vi "CAN_ParamShow.vi"(10 "DevType":u16, 11 "param":T2[](array[typedef]) {"ACR0" format="%x"}) -> ()   [LabVIEW 2011]
uses:
  VIs/Param.ctl
  VIs/Baud rate Self Define.ctl
panel:
  out "br_selfdef":T1={"BAUD"=0, "SJW"=1, "BRP"=1, "SAM"=0, "PHS2_SEL"=0, "SYN(nouse)"=1, "PRSEG"=1, "PHSEG1"=1, "PHSEG2"=1} {"PHSEG2" items=["CAN_BIT_1TQ"=1, "CAN_BIT_2TQ"=2, "CAN_BIT_3TQ"=3, "CAN_BIT_4TQ"=4, "CAN_BIT_5TQ"=5, "CAN_BIT_6TQ"=6, "CAN_BIT_7TQ"=7, "CAN_BIT_8TQ"=8]; "PHSEG1" items=["CAN_BIT_1TQ"=1, "CAN_BIT_2TQ"=2, "CAN_BIT_3TQ"=3, "CAN_BIT_4TQ"=4, "CAN_BIT_5TQ"=5, "CAN_BIT_6TQ"=6, "CAN_BIT_7TQ"=7, "CAN_BIT_8TQ"=8]; "PRSEG" items=["CAN_BIT_1TQ"=1, "CAN_BIT_2TQ"=2, "CAN_BIT_3TQ"=3, "CAN_BIT_4TQ"=4, "CAN_BIT_5TQ"=5, "CAN_BIT_6TQ"=6, "CAN_BIT_7TQ"=7, "CAN_BIT_8TQ"=8]; "PHS2_SEL" items=["由相位缓冲段1时间指定", "可编程"]; "SAM" items=["采样一次", "采样三次"]; "BRP" items=["1"=1, "2"=2, "3"=3, "4"=4, "5"=5, "6"=6, "7"=7, "8"=8, "9"=9, "10"=10, "11"=11, "12"=12, "13"=13, "14"=14, "15"=15, "16"=16, "17"=17, "18"=18, "19"=19, "20"=20, "21"=21, "22"=22, "23"=23, "24"=24, "25"=25, "26"=26, "27"=27, "28"=28, "29"=29, "30"=30, "31"=31, "32"=32, "33"=33, "34"=34, "35"=35, "36"=36, "37"=37, "38"=38, "39"=39, "40"=40, "41"=41, "42"=42, "43"=43, "44"=44, "45"=45, "46"=46, "47"=47, "48"=48, "49"=49, "50"=50, "51"=51, "52"=52, "53"=53, "54"=54, "55"=55, "56"=56, "57"=57, "58"=58, "59"=59, "60"=60, "61"=61, "62"=62, "63"=63, "64"=64]; "SJW" items=["1TQ"=1, "2TQ"=2, "3TQ"=3, "4TQ"=4]; "SYN(nouse)" items=["CAN_BIT_1TQ"=1]}
  out "Filter":u8(ring)=3 caption="滤波方式：" items=["接收所有类型"=1, "只收标准帧"=2, "只收扩展帧"=3]
  out "屏蔽码":u32=4294967295 caption="过滤屏蔽码:" format="%08x"
  out "验收码":u32=2147483648 caption="过滤验收码:" format="%08x"
  out "工作模式":u16(ring)=1 items=["正常工作", "仅监帧听模式", "自测模试（环回模式）"]
  out "br":u32(ring)=8 caption="波特率:" items=["Self Define", "5k bps", "10k bps", "20k bps", "40k bps", "50k bps", "80k bps", "100k bps", "125k bps", "200k bps", "250k bps", "400k bps", "500k bps", "666k bps", "800k bps", "1000k bps", "33.33k bps", "66.66k bps", "83.33k bps"]
  in  "channel":enum16{"通道1", "通道2"}(ring) caption="CAN通道"
  in  "ok":bool
  # "波特率设置"
  # "工作模式"
  # "滤波器"
  # "(HEX)"
  # "(HEX)"
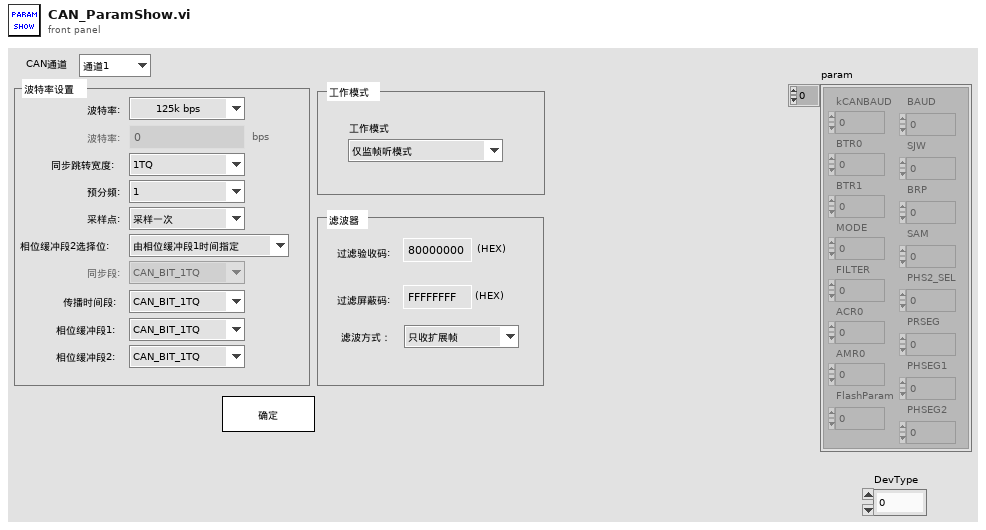
[diagram p1: front panel]
types:
  T1 = typedef "Baud rate Self Define.ctl" = cluster{"BAUD":u32, "SJW":u8, "BRP":u8, "SAM":u8, "PHS2_SEL":u8, "SYN(nouse)":u8, "PRSEG":u8, "PHSEG1":u8, "PHSEG2":u8}
  T2 = typedef "Param.ctl" = cluster{"kCANBAUD":u8, "BTR0":u8, "BTR1":u8, "MODE":u8, "FILTER":u8, "ACR0":u32, "AMR0":u32, "FlashParam":u32, "BAUD":u32, "SJW":u8, "BRP":u8, "SAM":u8, "PHS2_SEL":u8, "PRSEG":u8, "PHSEG1":u8, "PHSEG2":u8}
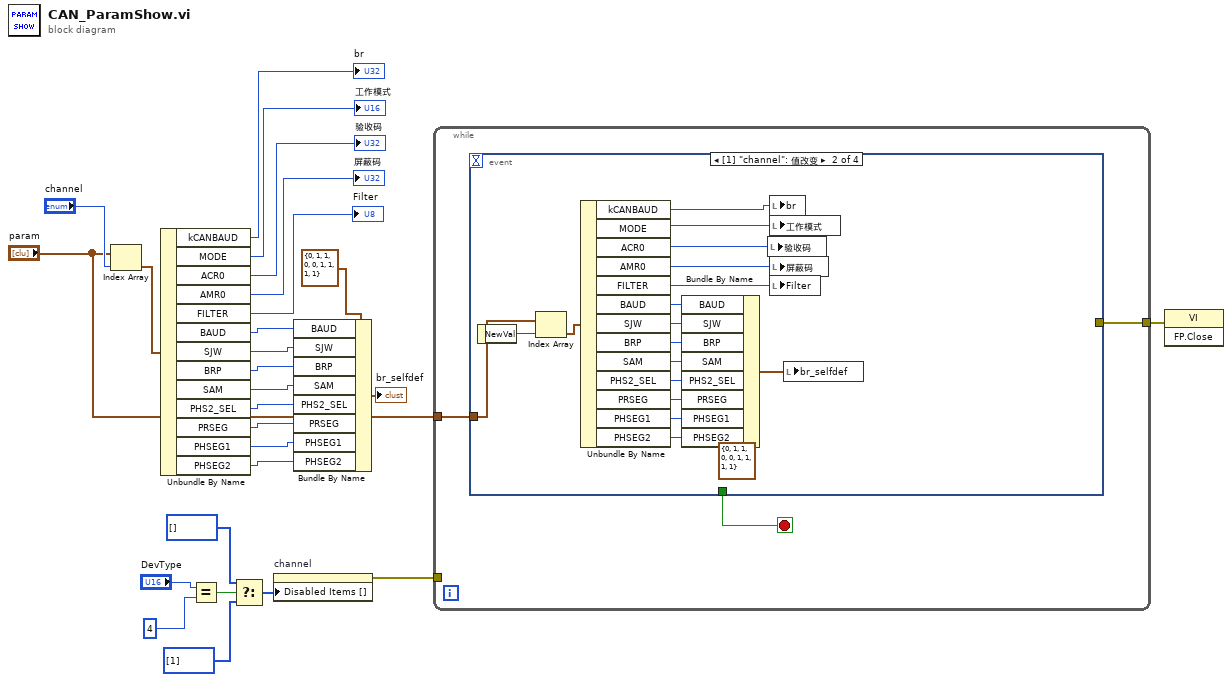
[diagram p0: block diagram]
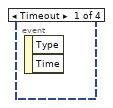
[diagram p2: hidden frame]
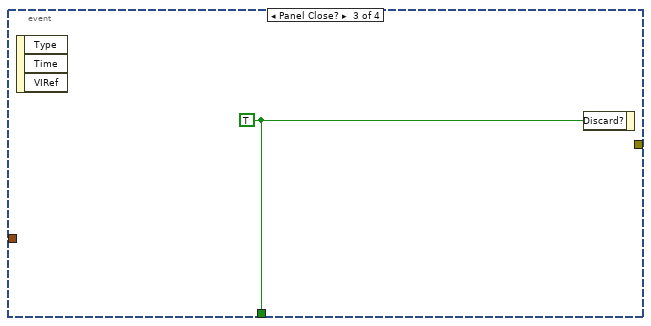
[diagram p3: hidden frame]
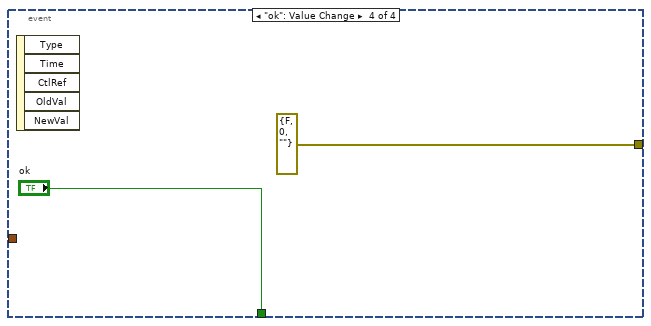
[diagram p4: hidden frame]
diagram:
  n1 = Index Array(array="param", index="channel") -> (element=w25:T2)
  n2 = Unbundle By Name(w25) -> ("kCANBAUD"=→"br":u8, "MODE"=→"工作模式":u8, "ACR0"=→"验收码":u32, "AMR0"=→"屏蔽码":u32, "FILTER"=→"Filter":u8, "BAUD"=w8:u32, "SJW"=w7:u8, "BRP"=w6:u8, "SAM"=w5:u8, "PHS2_SEL"=w4:u8, "PRSEG"=w3:u8, "PHSEG1"=w2:u8, "PHSEG2"=w1:u8)
  n3 = Equal?(x="DevType", y=u16 4) -> (x = y?=w21:bool)
  n4 = Select(t=i32[] [] ("禁用项[]"), s=w21, f=i32[] [1] ("禁用项[]")) -> (s? t:f=w18:i32[])
  n5 = property on="channel" class="Enum (严格)"("Disabled Items []"=w18) -> (error out=w17:errorcluster)  [unwired: 2 in, 1 out]
  n6 = Bundle By Name(cluster=T1 {"BAUD"=0, "SJW"=1, "BRP"=1, "SAM"=0, "PHS2_SEL"=0, "SYN(nouse)"=1, "PRSEG"=1, "PHSEG1"=1, "PHSEG2"=1} ("br_selfdef"), "BAUD"=w8, "SJW"=w7, "BRP"=w6, "SAM"=w5, "PHS2_SEL"=w4, "PRSEG"=w3, "PHSEG1"=w2, "PHSEG2"=w1) -> (→"br_selfdef":T1)
  n7 = while {
    tunnel: [w28] -> w26
    tunnel: "param" -> [w27]
    tunnel: w17 -> [_]
    stop <- w29 stop-if-true
    n8 = event shown="[1] \"channel\": 值改变" {
      selector: _ -> [_ _ _ _]
      dyn-events: _ -> [_ _ _ _]
      timeout: _ -> [_ _ _ _]
      tunnel: [_ _ w48 "ok"] -> w29
      tunnel: [_ _ _ errorcluster {"status"=FALSE, "code"=0, "source"=""} ("错误输入（无错误）")] -> w28
      tunnel: w27 -> [_ w47 _ _]
      event Timeout {
        n9 = event-data() -> ()  [unwired: 1 in, 2 out]
      }
      event "channel": Value Change {
        n10 = event-data() -> ("NewVal"=w46:enum16{"通道1", "通道2"})  [unwired: 1 in]
        n11 = Index Array(array=w47, index=w46) -> (element=w45:T2)
        n12 = Unbundle By Name(w45) -> ("kCANBAUD"=w44:u8, "MODE"=w43:u8, "ACR0"=w42:u32, "AMR0"=w41:u32, "FILTER"=w40:u8, "BAUD"=w38:u32, "SJW"=w31:u8, "BRP"=w32:u8, "SAM"=w33:u8, "PHS2_SEL"=w34:u8, "PRSEG"=w35:u8, "PHSEG1"=w36:u8, "PHSEG2"=w37:u8)
        n13 = Bundle By Name(cluster=T1 {"BAUD"=0, "SJW"=1, "BRP"=1, "SAM"=0, "PHS2_SEL"=0, "SYN(nouse)"=1, "PRSEG"=1, "PHSEG1"=1, "PHSEG2"=1} ("br_selfdef"), "BAUD"=w38, "SJW"=w31, "BRP"=w32, "SAM"=w33, "PHS2_SEL"=w34, "PRSEG"=w35, "PHSEG1"=w36, "PHSEG2"=w37) -> (w30:T1)
        n14 = local write "验收码"(w42) -> ()
        n15 = local write "br"(w44) -> ()
        n16 = local write "工作模式"(w43) -> ()
        n17 = local write "屏蔽码"(w41) -> ()
        n18 = local write "Filter"(w40) -> ()
        n19 = local write "br_selfdef"(w30) -> ()
      }
      event Panel Close? {
        w48 = TRUE ("放弃？")
        n20 = event-data() -> ()  [unwired: 1 in, 3 out]
        n21 = event-data("Discard?"=w48) -> ()  [unwired: 1 in, 1 out]
      }
      event "ok": Value Change {
        n22 = event-data() -> ()  [unwired: 1 in, 5 out]
      }
    }
  }
  n23 = invoke class="VI" method="FP.Close"(error in=w26) -> ()  [unwired: 2 in, 3 out]
